vi "Init.vi"(8 "error in (no error)":errorcluster, 11 "Cache Manager DVR in":refnum<class "Cache Manager.lvclass">) -> (0 "error out":errorcluster, 3 "Cache Manager DVR out":refnum<class "Cache Manager.lvclass">)   [LabVIEW 2020, in "Cache Manager.lvclass"]
uses:
  Cache Manager.lvclass
  Cache Manager.lvclass/Cache Manager.ctl
  Serializer/Serializable Message/Serializable Msg.lvclass
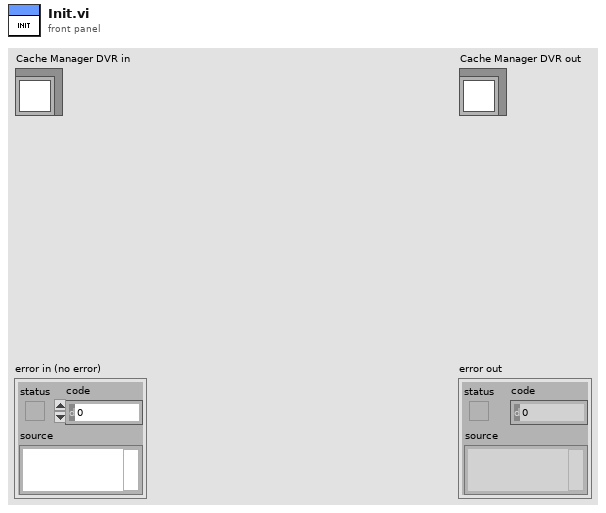
[diagram p1: front panel]
types:
  T1 = map{string, refnum<class "Serializable Msg.lvclass">}
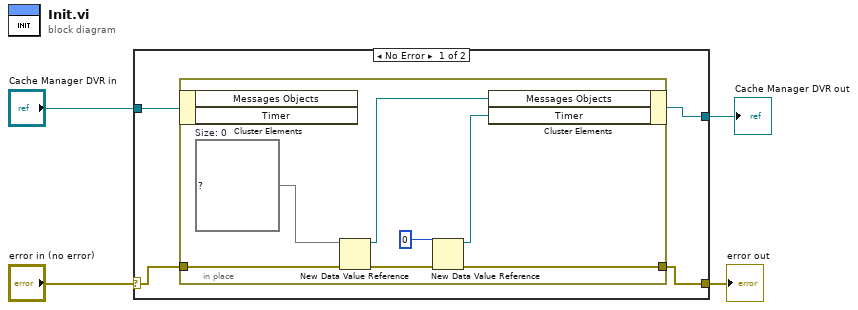
[diagram p0: block diagram]
diagram:
  n1 = case shown="No Error" "error in (no error)" {
    selector: "error in (no error)" -> [w6 w17]
    tunnel: [w5 w17] -> w3
    tunnel: [w7 w16] -> w1
    tunnel: "Cache Manager DVR in" -> [w8 w16]
    frame No Error {
      n2 = in-place "In Place Element Structure" {
        in-place-border: w6 -> [w13]
        in-place-border: [w11] -> w5
        w15 = T1 {}  # Size: 0
        n3 = in-place-cluster #1(w8) -> ()  [unwired: 2 out]
        n4 = New Data Value Reference(data value=w15, error in=w13) -> (data value reference=w14:refnum<data-value>, error out=w10:errorcluster)
        n5 = New Data Value Reference(data value=u32 0 ("start time"), error in=w10) -> (data value reference=w9:refnum<data-value>, error out=w11:errorcluster)
        n6 = in-place-cluster #1("Messages Objects"=w14, "Timer"=w9) -> (w7:refnum<class "Cache Manager.lvclass">)
      }
    }
    frame Error {
    }
  }
  "error out" <- w3
  "Cache Manager DVR out" <- w1
